vi "File.Async Mover, Assign Task.vi"(5 "Action":enum16{"Move", "Copy"}(ring), 6 "DestSuffix":string, 7 "Q Name":string="FileMover", 8 "error in":errorcluster, 9 "Destination":path, 11 "Source":path) -> (0 "error out":errorcluster)   [LabVIEW 2018]
uses:
  File.Async Mover Move Task Item.ctl
  <vilib>/KATE/Queues/Queue Utils.lvlib
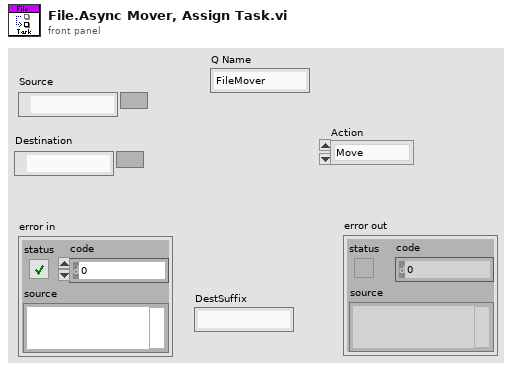
[diagram p1: front panel]
types:
  T1 = typedef "File.Async Mover Move Task Item.ctl" = cluster{"Source":path, "DestDir":path, "DestSuffix":string, "Action":enum16{"Move", "Copy"}}
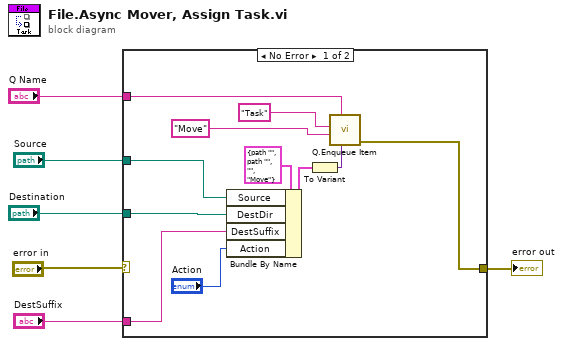
[diagram p0: block diagram]
diagram:
  n1 = case shown="No Error" "error in" {
    selector: "error in" -> [_ w18]
    tunnel: "Q Name" -> [w17 _]
    tunnel: "Source" -> [w13 _]
    tunnel: "Destination" -> [w12 _]
    tunnel: [w11 w18] -> w3
    tunnel: "DestSuffix" -> [w8 _]
    frame No Error {
      n2 = Bundle By Name(cluster=T1 {"Source"=path "", "DestDir"=path "", "DestSuffix"="", "Action"=enum."Move"}, "Source"=w13, "DestDir"=w12, "DestSuffix"=w8, "Action"="Action") -> (w14:T1)
      n3 = To Variant(anything=w14) -> (Variant=w15:variant)
      n4 = call <vilib>:"Q.Enqueue Item.vi"("Data1"=w15, "Q Name"=w17, "Sub"="Move" ("Task Name"), "Cmd"="Task" ("Task Name")) -> ("error out"=w11:errorcluster)  [unwired: 6 in, 1 out]
    }
    frame Error {
    }
  }
  "error out" <- w3
